vi "IO Mapping.vi"(8 "error in (no error)":errorcluster, 11 "Configuration in":refnum<class "Configuration.lvclass">) -> (0 "error out":errorcluster, 3 "Configuration out":refnum<class "Configuration.lvclass">)   [LabVIEW 2026, in "Hardware.lvlib" / "HW Configuration.lvclass"]
uses:
  HW Configuration.lvclass
  Extensible-Config-Dialog/Configuration.lvclass
  HW Configuration.lvclass/HW Configuration.ctl
panel:
  in  "IO Mapping":T1
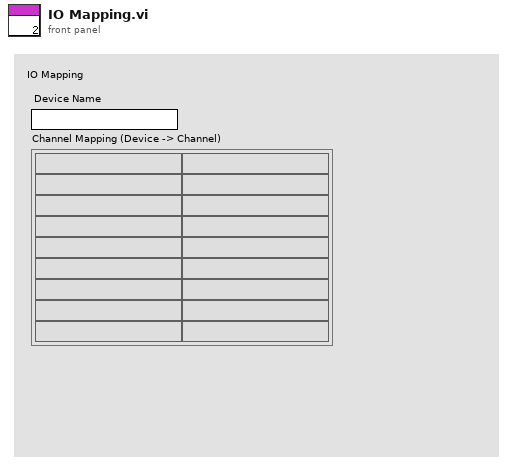
[diagram p1: front panel]
types:
  T1 = cluster{"Device Name":string, "Channel Mapping (Device -> Channel)":string[][]}
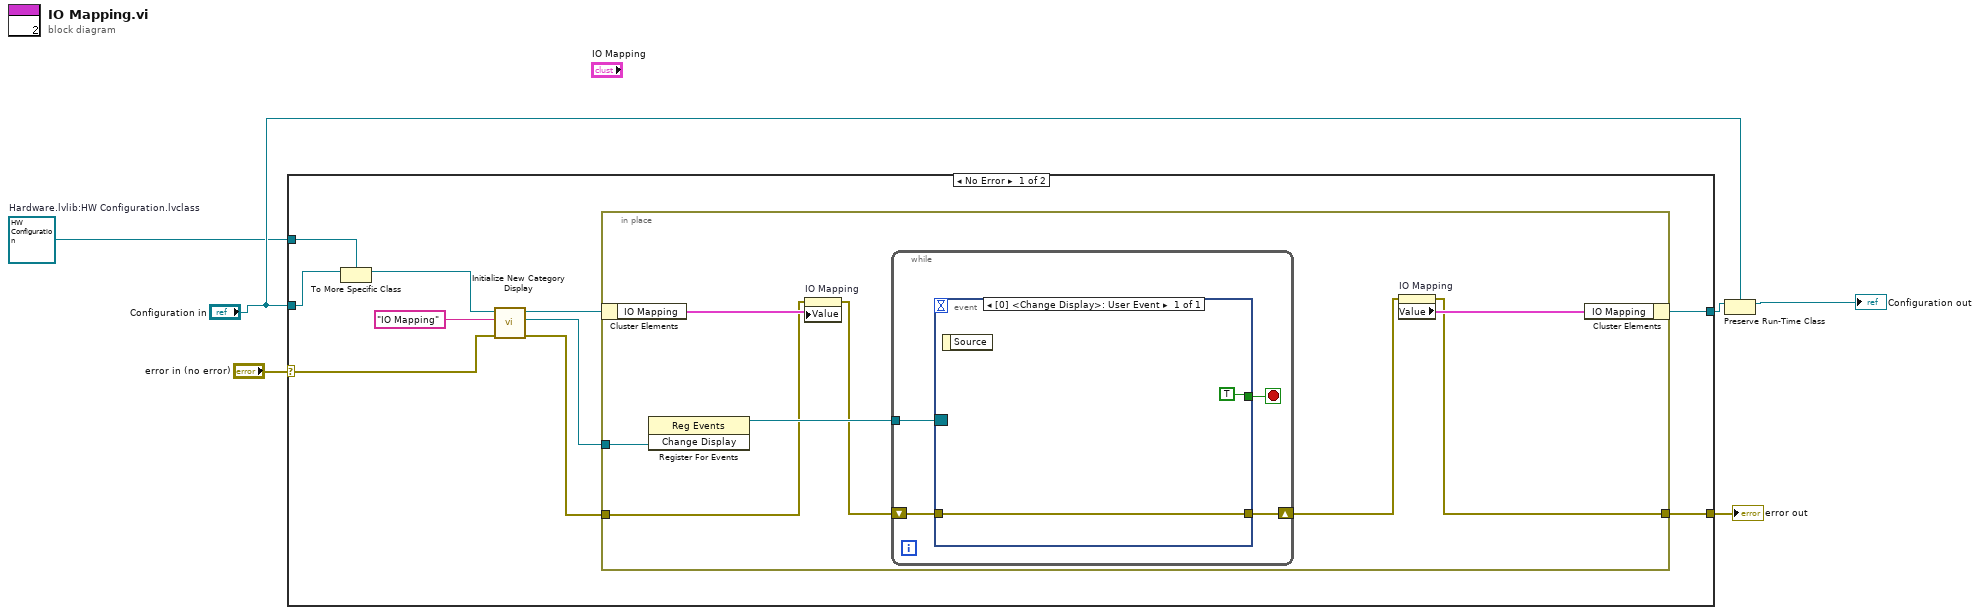
[diagram p0: block diagram]
diagram:
  w1 = refnum<class "HW Configuration.lvclass"> refnum  # Hardware.lvlib:HW Configuration.lvclass
  n1 = case shown="No Error" "error in (no error)" {
    selector: "error in (no error)" -> [w13 w32]
    tunnel: [w8 w31] -> w3
    tunnel: [w7 w32] -> w6
    tunnel: "Configuration in" -> [w12 w31]
    tunnel: w1 -> [w10 _]
    frame No Error {
      n2 = To More Specific Class(target class=w10, reference=w12) -> (specific class reference=w11:refnum<class "HW Configuration.lvclass">)  [unwired: 1 in, 1 out]
      n3 = call "Initialize New Category Display.vi"("error in (no error)"=w13, "Name to Display"="IO Mapping", "Configuration in"=w11) -> ("error out"=w15:errorcluster, "Change Display"=w16:refnum<user-event>, "Configuration Out"=w9:refnum<class "HW Configuration.lvclass">)  [unwired: 6 in]
      n4 = in-place {
        in-place-border: w16 -> [w24]
        in-place-border: w15 -> [w21]
        in-place-border: [w17] -> w7
        n5 = in-place-cluster #1(w9) -> ("IO Mapping"=w22:T1)
        n6 = register-events(w24) -> (reference out=w23:refnum<event-registration>)  [unwired: 2 in, 1 out]
        n7 = property on="IO Mapping" class="Clust (strict)"(error in=w21, "Value"=w22) -> (error out=w20:errorcluster)  [unwired: 1 in, 1 out]
        n8 = while {
          tunnel: w23 -> [w27]
          shift-right: [w26] -> w18
          shift-left: w20 -> [w25]
          stop <- w28 stop-if-true
          n9 = event shown="[0] <Change Display>: User Event" {
            selector: w27 -> [_]
            dyn-events: _ -> [_]
            timeout: _ -> [_]
            tunnel: [TRUE] -> w28
            tunnel: [w29] -> w26
            tunnel: w25 -> [w29]
            event User Event {
              n10 = event-data() -> ()  [unwired: 1 in, 1 out]
            }
          }
        }
        n11 = property on="IO Mapping" class="Clust (strict)"(error in=w18) -> (error out=w17:errorcluster, "Value"=w19:T1)  [unwired: 1 in, 1 out]
        n12 = in-place-cluster #1("IO Mapping"=w19) -> (w8:refnum<class "HW Configuration.lvclass">)
      }
    }
    frame Error {
    }
  }
  "error out" <- w6
  n13 = Preserve Run-Time Class(object in=w3, 2:"Configuration in") -> (object out=→"Configuration out":refnum<class "Configuration.lvclass">)  [unwired: 1 in, 1 out]
